vi "lvoption.vi"   [LabVIEW 2020]
uses:
  <vilib>/Wiresmith Technology/G CLI/Argument Parser/Option Class/Option Configuration.ctl
  <vilib>/Wiresmith Technology/G CLI/Argument Parser/Option Class/Argument Type.ctl
  <vilib>/Utility/error.llb/DialogType.ctl
  094f6021-4ef8-4573-82ce-a7b4949f6c5c.vi
  35111923-3b9e-4c36-b72b-79289da6bcaf.vi
  0b828e9d-cbba-40c4-b017-a79c080be190.vi
  6795289f-0a04-455c-a499-a5e59a361415.vi
  <resource>/dialog/lvconfig.llb/LV Config Read String.vi
  <resource>/dialog/lvconfig.llb/LV Config Write String.vi
  <resource>/dialog/lvconfig.llb/LV Config Write Boolean.vi
  <resource>/dialog/lvconfig.llb/LV Config Write Numeric (I32).vi
  <vilib>/Comparison/Equal/Equal Functor/Equal Functor.lvclass
  <vilib>/Wiresmith Technology/G CLI/CLI Class/CLI.lvclass
  <vilib>/Wiresmith Technology/G CLI/Argument Parser/Option Set Class/Option Set.lvclass
  <vilib>/Wiresmith Technology/G CLI/Argument Parser/Option Class/Option.lvclass
  <resource>/dialog/lvconfig.llb/LV Config Write Color.vi
  <resource>/dialog/lvconfig.llb/LV Config Write Pathlist.vi
types:
  T1 = cluster{"VerboseMode":bool, "Operation":string, "Key":string}
  T2 = enum32{"Invalid", "Standard", "Closed", "Hidden", "Minimized", "Maximized"}
  T3 = typedef "Option Parser.lvlib/Option.lvclass/Option Configuration.ctl" = cluster{"Option Type":T4, "Option Labels":string[], "Key":string, "Description":string, "Required":bool, "Default Value":string}
  T4 = typedef "Option Parser.lvlib/Option.lvclass/Argument Type.ctl" = enum16{"flag", "value"}
  T5 = typedef "DialogType.ctl" = u16
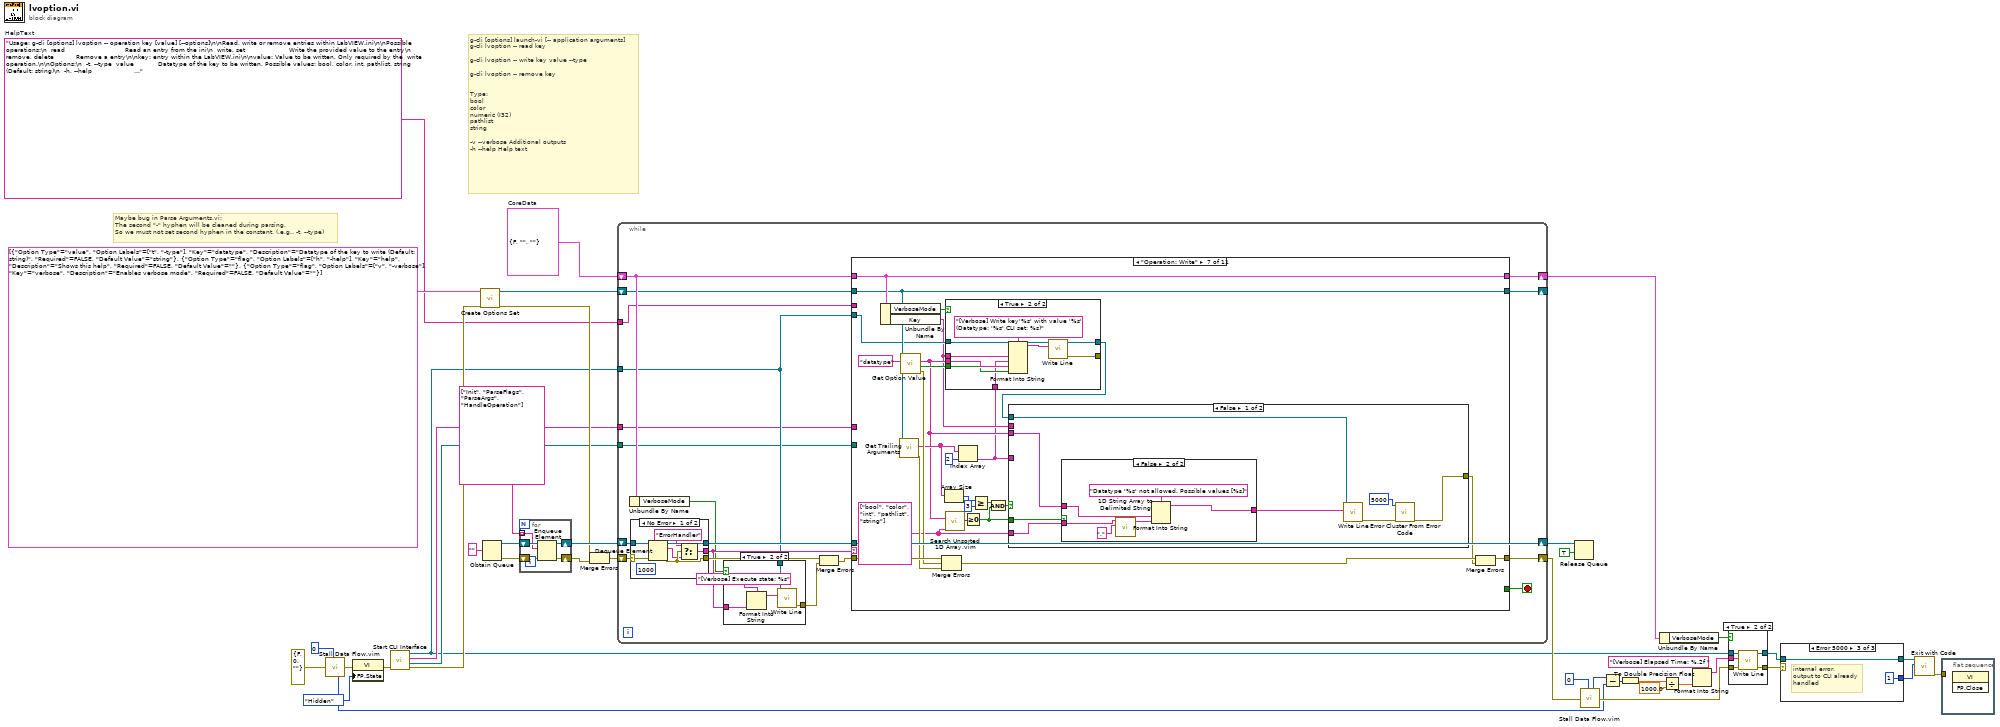
[diagram p0: block diagram]
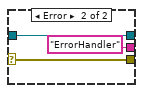
[diagram p4: hidden frame]
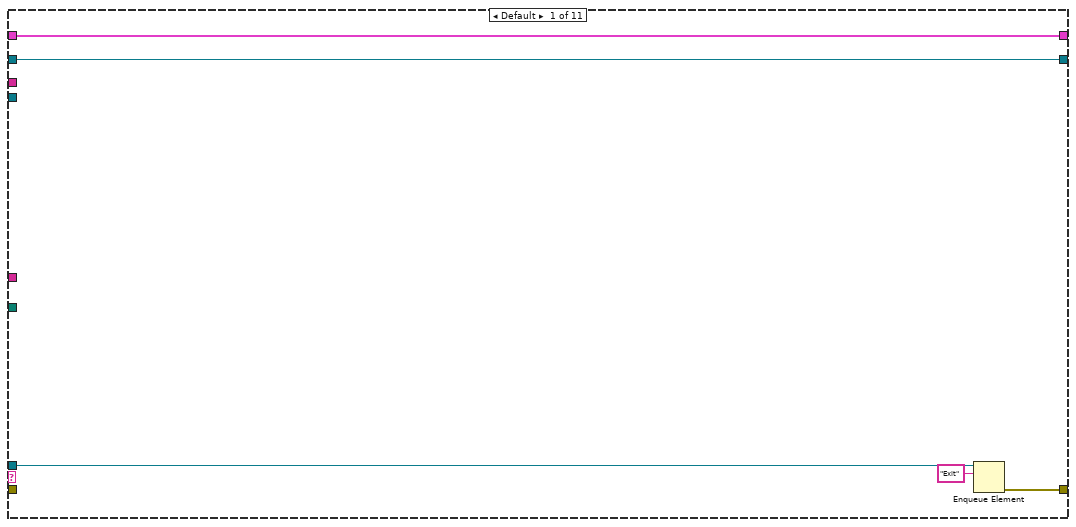
[diagram p5: hidden frame]
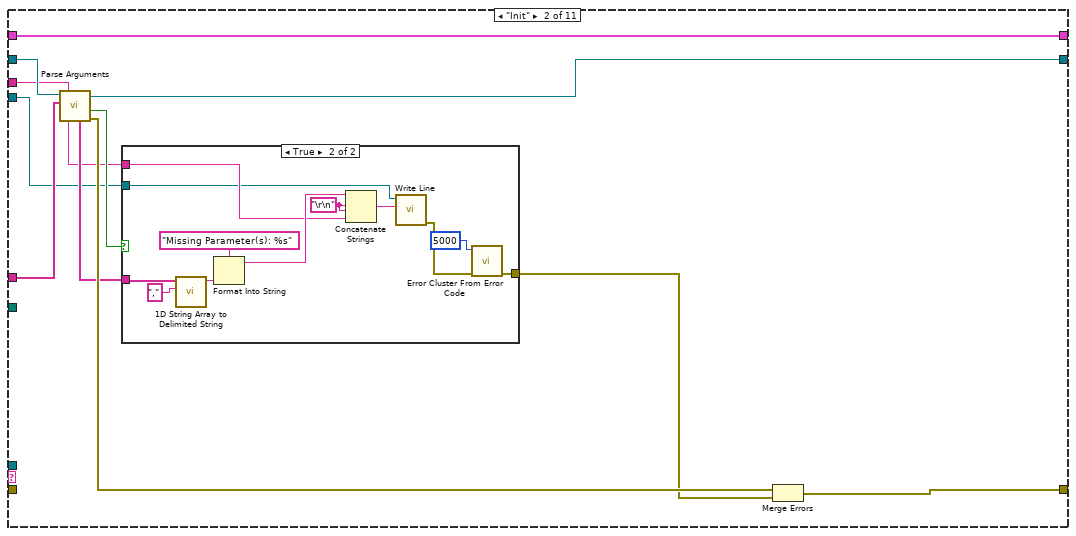
[diagram p6: hidden frame]
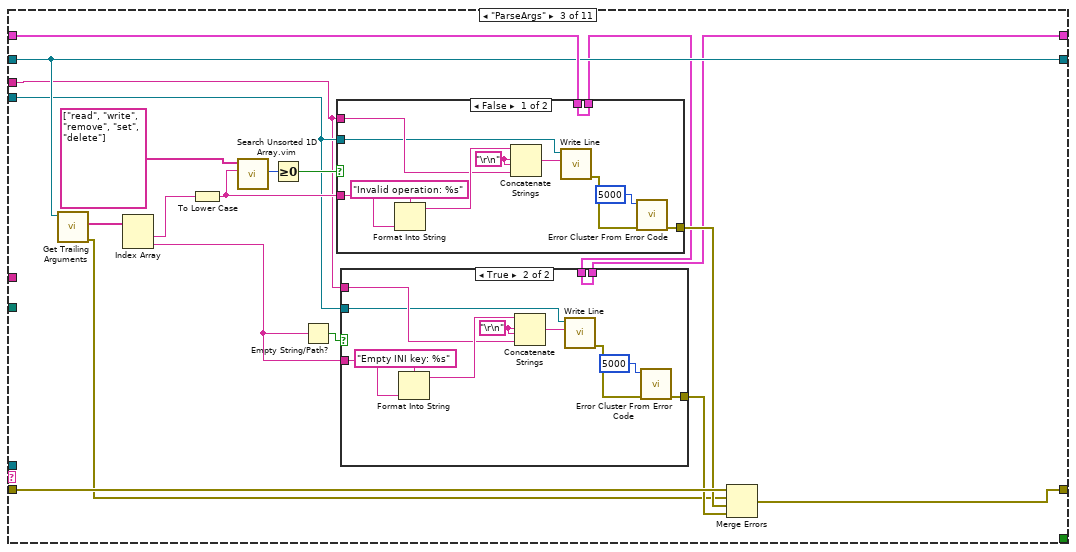
[diagram p8: hidden frame]
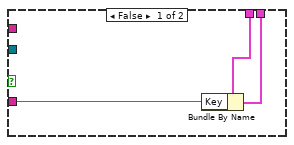
[diagram p9: hidden frame]
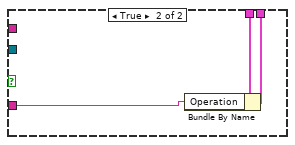
[diagram p10: hidden frame]
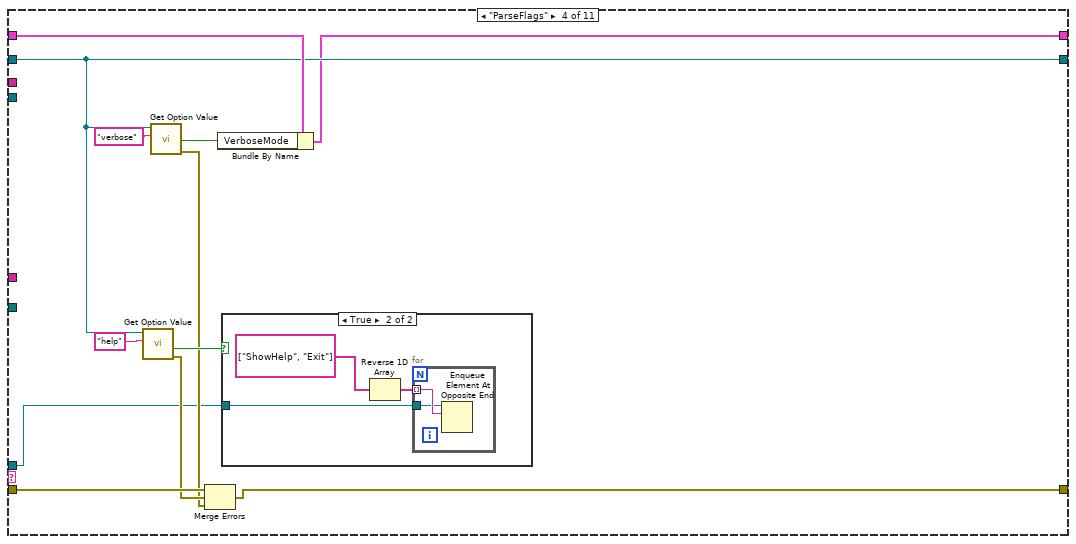
[diagram p11: hidden frame]
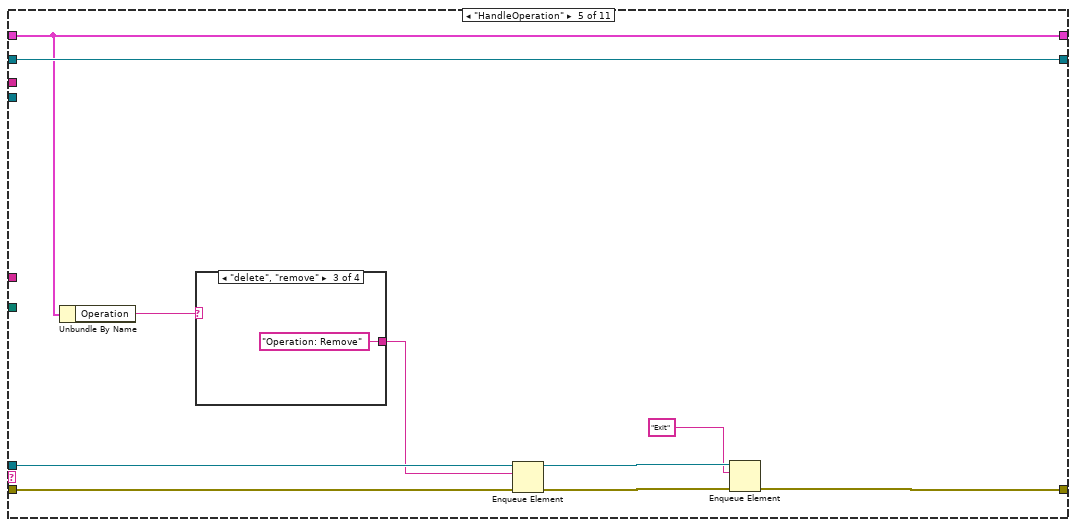
[diagram p13: hidden frame]
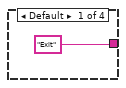
[diagram p14: hidden frame]
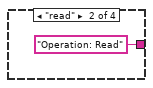
[diagram p15: hidden frame]
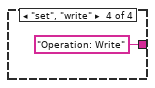
[diagram p16: hidden frame]
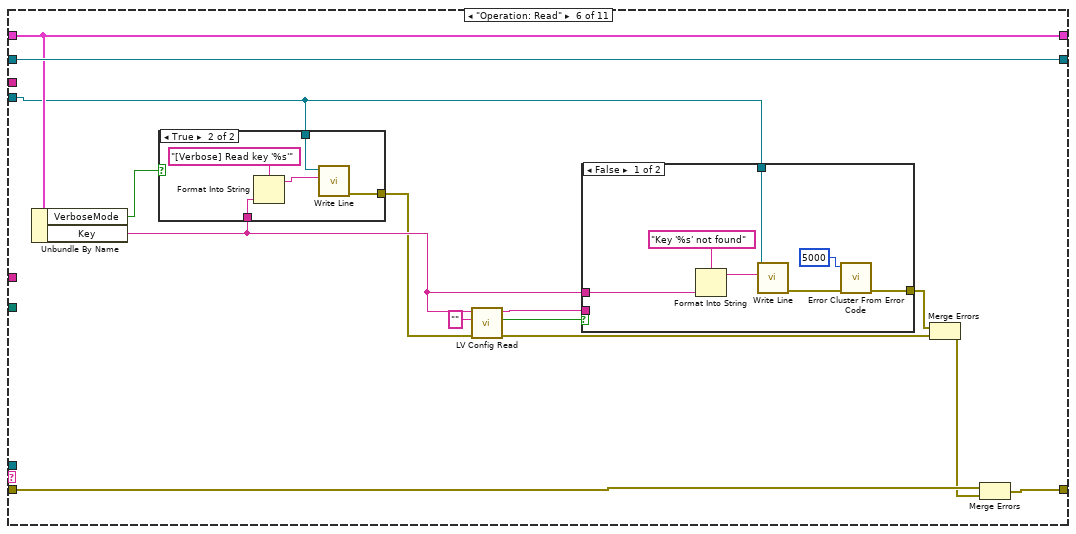
[diagram p17: hidden frame]
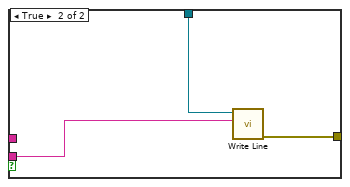
[diagram p19: hidden frame]
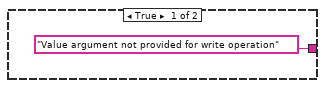
[diagram p20: hidden frame]
diagram:
  w1 = "Usage: g-cli [options] lvoption -- operation key [value] [--options]\n\nRead, write or remove entries within LabVIEW.ini\n\nPossible operations:\n  read                              Read an entry from the ini\n  write, set                      Write the provided value to the entry\n  remove, delete           Remove a entry\n\nkey: entry within the LabVIEW.ini\n\nvalue: Value to be written. Only required by the  write operation.\n\nOptions:\n  -t, --type  value            Datatype of the key to be written. Possible values: bool, color, int, pathlist, string (Default: string)\n  -h, --help                      Shows this help.\n  -v, --verbose                 Enables verbose mode."  # HelpText
  w14 = T1 {"VerboseMode"=FALSE, "Operation"="", "Key"=""}  # CoreData
  # "Maybe bug in Parse Arguments.vi: \nThe second \"-\" hyphen will be cleaned during parsing.\nSo we must not set second hyphen in the constant. (.e.g., -t, --type)"
  # "g-cli [options] launch-vi [-- application arguments]\ng-cli lvoption -- read key\n\ng-cli lvoption -- write key value --type \n\ng-cli lvoption -- remove key\n\n\nType:\nbool\ncolor\nnumeric (I32)\npathlist\nstring\n\n-v --verbose Additional outputs\n-h --help Help text"
  n1 = call "Stall Data Flow.vim"("value in"=errorcluster {"status"=FALSE, "code"=0, "source"=""} ("error in (no error)"), "milliseconds to wait"=u32 0) -> ("millisecond timer value"=w30:u32, "value out"=w37:errorcluster)
  n2 = property class="VI"(error in=w37, "FP.State"=T2."Hidden" ("Front Panel Window:State")) -> (error out=w36:errorcluster)  [unwired: 1 in, 1 out]
  n3 = call <vilib>:"Start CLI Interface.vi"("error in (no error)"=w36) -> ("error out"=w41:errorcluster, "Working Directory"=w7:path, "Custom Parameters"=w8:string[], "CLI out"=w5:refnum<class "CLI.lvclass">)  [unwired: 7 in]
  n4 = call <vilib>:"Create Options Set.vi"("error in (no error)"=w41, "Options"=T3[] [{"Option Type"=enum."value", "Option Labels"=["t", "-type"], "Key"="datatype", "Description"="Datatype of the key to write (Default: string)", "Required"=FALSE, "Default Value"="string"}, {"Option Type"=enum."flag", "Option Labels"=["h", "-help"], "Key"="help", "Description"="Shows this help", "Required"=FALSE, "Default Value"=""}, {"Option Type"=enum."flag", "Option Labels"=["v", "-verbose"], "Key"="verbose", "Description"="Enables verbose mode", "Required"=FALSE, "Default Value"=""}]) -> ("error out"=w10:errorcluster, "Option Set out"=w12:refnum<class "Option Set.lvclass">)  [unwired: 8 in]
  n5 = Obtain Queue(element data type="") -> (queue out=w19:refnum<queue>, error out=w16:errorcluster)  [unwired: 4 in, 1 out]
  n6 = for {
    shift-right: [w45] -> w17
    shift-left: w19 -> [w46]
    shift-right: [w43] -> w11
    shift-left: w16 -> [w44]
    tunnel: string[] ["Init", "ParseFlags", "ParseArgs", "HandleOperation"] -> [w42] mode=indexing
    n7 = Enqueue Element(queue=w46, element=w42, error in (no error)=w44) -> (queue out=w45:refnum<queue>, error out=w43:errorcluster)  [unwired: 1 in, 1 out]
  }
  n8 = Merge Errors(w10, w11) -> (w9:errorcluster)
  n9 = while {
    shift-right: [w61] -> w4
    shift-left: w14 -> [w56]
    shift-right: [w59] -> w6
    shift-left: w9 -> [w63]
    shift-right: [w58] -> w15
    shift-left: w17 -> [w64]
    tunnel: w5 -> [w54]
    tunnel: w8 -> [w49]
    tunnel: w7 -> [w50]
    tunnel: w1 -> [w48]
    shift-right: [w47] -> _
    shift-left: w12 -> [w53]
    stop <- w60 stop-if-true
    n10 = Unbundle By Name(w56) -> ("VerboseMode"=w55:bool)
    n11 = case shown="No Error" w63 {
      selector: w63 -> [w75 w79]
      tunnel: w64 -> [w76 w78]
      tunnel: [w71 "ErrorHandler"] -> w57
      tunnel: [w73 w79] -> w62
      tunnel: [w74 w78] -> w58
      frame No Error {
        (unwired) 1000 ("timeout in ms (-1)")
        n12 = Dequeue Element(queue=w76, error in (no error)=w75) -> (queue out=w74:refnum<queue>, element=w72:string, error out=w73:errorcluster)  [unwired: 1 in, 1 out]
        n13 = Select(t="ErrorHandler", s=w73, f=w72) -> (s? t:f=w71:string)
      }
      frame Error {
      }
    }
    n14 = case shown="True" w55 {
      tunnel: w57 -> [_ w69]
      tunnel: w54 -> [_ w66]
      tunnel: [_ w65] -> w51
      frame False {
      }
      frame True {
        n15 = Format Into String(format string="[Verbose] Execute state: %s", w69) -> (resulting string=w67:string)  [unwired: 2 in, 1 out]
        n16 = call <vilib>:"Write Line.vi"("Text to Write"=w67, "CLI in"=w66) -> ("error out"=w65:errorcluster)  [unwired: 8 in, 1 out]
      }
    }
    n17 = Merge Errors(w62, w51) -> (w52:errorcluster)
    n18 = case shown="\"Operation: Write\"" w57 {
      tunnel: w52 -> [_ _ w125 w163 w178 w197 w239 w300 _ w329 w332]
      tunnel: [w84 w95 w114 w155 w180 w198 w236 w305 w326 w330 w334] -> w61
      tunnel: w56 -> [w84 w95 w126 w166 w180 w198 w236 w305 w326 w330 w334]
      tunnel: [_ _ _ _ _ _ _ _ _ TRUE TRUE] -> w60
      tunnel: [w82 w87 w117 w160 w172 w196 w227 w307 w322 w329 w332] -> w59
      tunnel: w58 -> [w83 _ _ w156 w177 _ _ _ _ _ _]
      tunnel: w54 -> [_ w88 w113 _ _ w188 w224 w302 w324 _ _]
      tunnel: w53 -> [w80 w94 w124 w161 w181 w199 w234 w308 w325 w327 w331]
      tunnel: w50 -> [_ _ _ _ _ _ _ _ _ _ _]
      tunnel: w49 -> [_ w93 _ _ _ _ _ _ _ _ _]
      tunnel: w48 -> [_ w89 w112 _ _ _ _ _ w323 _ _]
      tunnel: [w80 w85 w124 w161 w181 w199 w234 w308 w325 w327 w331] -> w47
      frame Default {
        n19 = Enqueue Element(queue=w83, element="Exit") -> (error out=w82:errorcluster)  [unwired: 2 in, 2 out]
      }
      frame "Init" {
        n20 = call <vilib>:"Parse Arguments.vi"("Arguments"=w93, "Option Set in"=w94) -> ("error out"=w92:errorcluster, "Missing Options"=w91:bool, "Option Set out"=w85:refnum<class "Option Set.lvclass">, "Missing Option Keys"=w90:string[])  [unwired: 6 in]
        n21 = case shown="True" w91 {
          tunnel: w90 -> [_ w106]
          tunnel: w89 -> [_ w101]
          tunnel: w88 -> [_ w99]
          tunnel: [_ w96] -> w86
          frame False {
          }
          frame True {
            w103 = "\r\n"
            n22 = call <vilib>:"1D String Array to Delimited String.vi"("delimiter"=",", "string array"=w106) -> ("delimited string"=w104:string)  [unwired: 9 in]
            n23 = Format Into String(format string="Missing Parameter(s): %s", w104) -> (resulting string=w102:string)  [unwired: 2 in, 1 out]
            n24 = Concatenate Strings(w102, w103, w103, w101) -> (w100:string)
            n25 = call <vilib>:"Write Line.vi"("Text to Write"=w100, "CLI in"=w99) -> ("error out"=w97:errorcluster)  [unwired: 8 in, 1 out]
            n26 = call <vilib>:"Error Cluster From Error Code.vi"("error in (no error)"=w97, "error code (0)"=5000) -> ("error out"=w96:errorcluster)  [unwired: 7 in]
          }
        }
        n27 = Merge Errors(w92, w86) -> (w87:errorcluster)
      }
      frame "ParseArgs" {
        n28 = call <vilib>:"Get Trailing Arguments.vi"("Option Set in"=w124) -> ("error out"=w108:errorcluster, "Arguments"=w123:string[])  [unwired: 8 in, 1 out]
        n29 = Index Array(array=w123) -> (element #1=w122:string, element #2=w111:string)  [unwired: 2 in]
        n30 = To Lower Case(string=w122) -> (all lower case string=w118:string)
        n31 = call "Search Unsorted 1D Array.vim"("element"=w118, "unsorted 1D array"=string[] ["read", "write", "remove", "set", "delete"]) -> ("index of element"=w120:i32)  [unwired: 9 in]
        n32 = Greater Or Equal To 0?(x=w120) -> (x >= 0?=w119:bool)
        n33 = Empty String/Path?(string/path=w111) -> (empty?=w110:bool)
        n34 = case shown="False" w119 {
          tunnel: w112 -> [w148 _]
          tunnel: w113 -> [w146 _]
          tunnel: [w143 _] -> w116
          tunnel: w126 -> [w142 w154]
          tunnel: w118 -> [w141 w153]
          tunnel: [w142 w152] -> w115
          frame False {
            w150 = "\r\n"
            n35 = Format Into String(format string="Invalid operation: %s", w141) -> (resulting string=w149:string)  [unwired: 2 in, 1 out]
            n36 = Concatenate Strings(w149, w150, w150, w148) -> (w147:string)
            n37 = call <vilib>:"Write Line.vi"("Text to Write"=w147, "CLI in"=w146) -> ("error out"=w144:errorcluster)  [unwired: 8 in, 1 out]
            n38 = call <vilib>:"Error Cluster From Error Code.vi"("error in (no error)"=w144, "error code (0)"=5000) -> ("error out"=w143:errorcluster)  [unwired: 7 in]
          }
          frame True {
            n39 = Bundle By Name(cluster=w154, "Operation"=w153) -> (w152:T1)
          }
        }
        n40 = case shown="True" w110 {
          tunnel: w112 -> [_ w137]
          tunnel: w113 -> [_ w135]
          tunnel: [_ w132] -> w109
          tunnel: w115 -> [w129 w131]
          tunnel: w111 -> [w128 w130]
          tunnel: [w127 w131] -> w114
          frame False {
            n41 = Bundle By Name(cluster=w129, "Key"=w128) -> (w127:T1)
          }
          frame True {
            w139 = "\r\n"
            n42 = Format Into String(format string="Empty INI key: %s", w130) -> (resulting string=w138:string)  [unwired: 2 in, 1 out]
            n43 = Concatenate Strings(w138, w139, w139, w137) -> (w136:string)
            n44 = call <vilib>:"Write Line.vi"("Text to Write"=w136, "CLI in"=w135) -> ("error out"=w133:errorcluster)  [unwired: 8 in, 1 out]
            n45 = call <vilib>:"Error Cluster From Error Code.vi"("error in (no error)"=w133, "error code (0)"=5000) -> ("error out"=w132:errorcluster)  [unwired: 7 in]
          }
        }
        n46 = Merge Errors(w125, w108, w116, w109) -> (w117:errorcluster)
      }
      frame "ParseFlags" {
        n47 = call <vilib>:"Get Option Value.vi"("Option Key"="help", "Option Set in"=w161) -> ("error out"=w159:errorcluster, "Set"=w164:bool)  [unwired: 6 in, 2 out]
        n48 = call <vilib>:"Get Option Value.vi"("Option Key"="verbose", "Option Set in"=w161) -> ("error out"=w158:errorcluster, "Set"=w157:bool)  [unwired: 6 in, 2 out]
        n49 = Merge Errors(w163, w159, w158) -> (w160:errorcluster)
        n50 = Bundle By Name(cluster=w166, "VerboseMode"=w157) -> (w155:T1)
        n51 = case shown="True" w164 {
          tunnel: w156 -> [_ w168]
          frame False {
          }
          frame True {
            n52 = Reverse 1D Array(array=string[] ["ShowHelp", "Exit"]) -> (reversed array=w167:string[])
            n53 = for {
              tunnel: w167 -> [w171] mode=indexing
              tunnel: w168 -> [w170]
              n54 = Enqueue Element At Opposite End(queue=w170, element=w171) -> ()  [unwired: 2 in, 3 out]
            }
          }
        }
      }
      frame "HandleOperation" {
        n55 = Unbundle By Name(w180) -> ("Operation"=w179:string)
        n56 = case shown="\"delete\", \"remove\"" w179 {
          tunnel: ["Exit" "Operation: Read" "Operation: Remove" "Operation: Write"] -> w176
          frame Default {
          }
          frame "read" {
          }
          frame "delete", "remove" {
          }
          frame "set", "write" {
          }
        }
        n57 = Enqueue Element(queue=w177, element=w176, error in (no error)=w178) -> (queue out=w174:refnum<queue>, error out=w175:errorcluster)  [unwired: 1 in, 1 out]
        n58 = Enqueue Element(queue=w174, element="Exit", error in (no error)=w175) -> (error out=w172:errorcluster)  [unwired: 1 in, 2 out]
      }
      frame "Operation: Read" {
        n59 = Unbundle By Name(w198) -> ("VerboseMode"=w189:bool, "Key"=w187:string)
        n60 = case shown="True" w189 {
          tunnel: w188 -> [_ w204]
          tunnel: w187 -> [_ w201]
          tunnel: [_ w200] -> w186
          frame False {
          }
          frame True {
            n61 = Format Into String(format string="[Verbose] Read key '%s'", w201) -> (resulting string=w203:string)  [unwired: 2 in, 1 out]
            n62 = call <vilib>:"Write Line.vi"("Text to Write"=w203, "CLI in"=w204) -> ("error out"=w200:errorcluster)  [unwired: 8 in, 1 out]
          }
        }
        n63 = call-poly <resource>:"LV Config Read.vi"("error in"=w186, "default value"="", "key"=w187) -> ("error out"=w195:errorcluster, "found?"=w193:bool, "value"=w190:string)  [unwired: 2 in]
        n64 = case shown="False" w193 {
          tunnel: w187 -> [w207 _]
          tunnel: [w206 w213] -> w191
          tunnel: w188 -> [w205 w214]
          tunnel: w190 -> [_ w212]
          frame False {
            n65 = Format Into String(format string="Key '%s' not found", w207) -> (resulting string=w209:string)  [unwired: 2 in, 1 out]
            n66 = call <vilib>:"Write Line.vi"("Text to Write"=w209, "CLI in"=w205) -> ("error out"=w210:errorcluster)  [unwired: 8 in, 1 out]
            n67 = call <vilib>:"Error Cluster From Error Code.vi"("error in (no error)"=w210, "error code (0)"=5000) -> ("error out"=w206:errorcluster)  [unwired: 7 in]
          }
          frame True {
            n68 = call <vilib>:"Write Line.vi"("Text to Write"=w212, "CLI in"=w214) -> ("error out"=w213:errorcluster)  [unwired: 8 in, 1 out]
          }
        }
        n69 = Merge Errors(w191, w195) -> (w192:errorcluster)
        n70 = Merge Errors(w197, w192) -> (w196:errorcluster)
      }
      frame "Operation: Write" {
        w218 = string[] ["bool", "color", "int", "pathlist", "string"]
        n71 = Unbundle By Name(w236) -> ("VerboseMode"=w235:bool, "Key"=w216:string)
        n72 = call <vilib>:"Get Trailing Arguments.vi"("Option Set in"=w234) -> ("error out"=w230:errorcluster, "Arguments"=w228:string[])  [unwired: 8 in, 1 out]
        n73 = call <vilib>:"Get Option Value.vi"("Option Key"="datatype", "Option Set in"=w234) -> ("error out"=w229:errorcluster, "Set"=w237:bool, "Value"=w221:string)  [unwired: 6 in, 1 out]
        n74 = Merge Errors(w239, w229, w230) -> (w231:errorcluster)
        n75 = Array Size(array=w228) -> (size(s)=w233:i32)
        n76 = call "Search Unsorted 1D Array.vim"("element"=w221, "unsorted 1D array"=w218) -> ("index of element"=w222:i32)  [unwired: 9 in]
        n77 = Index Array(array=w228, index=2) -> (element=w215:string)
        n78 = case shown="True" w235 {
          tunnel: w221 -> [_ w299]
          tunnel: w237 -> [_ w298]
          tunnel: w224 -> [w290 w295]
          tunnel: [w290 w294] -> w225
          tunnel: [_ w293] -> _
          tunnel: w216 -> [_ w292]
          tunnel: w215 -> [_ w291]
          frame False {
          }
          frame True {
            n79 = Format Into String(format string="[Verbose] Write key'%s' with value '%s' (Datatype: '%s' CLI set: %s)", w292, w291, w299, w298) -> (resulting string=w296:string)  [unwired: 2 in, 1 out]
            n80 = call <vilib>:"Write Line.vi"("Text to Write"=w296, "CLI in"=w295) -> ("error out"=w293:errorcluster, "CLI out"=w294:refnum<class "CLI.lvclass">)  [unwired: 8 in]
          }
        }
        n81 = Greater Or Equal To 0?(x=w222) -> (x >= 0?=w220:bool)
        n82 = Greater Or Equal?(x=w233, y=3) -> (x >= y?=w219:bool)
        n83 = Compound Arithmetic op=AND(w219, w220) -> (w223:bool)
        n84 = case shown="False" w223 {
          tunnel: w225 -> [w244 w256]
          tunnel: [w243 w257] -> w226
          tunnel: w221 -> [w241 w258]
          tunnel: w220 -> [w242 _]
          tunnel: w218 -> [w240 _]
          tunnel: w216 -> [_ w259]
          tunnel: w215 -> [_ w255]
          frame False {
            n85 = case shown="False" w242 {
              tunnel: ["Value argument not provided for write operation" ("format string") w254] -> w245
              tunnel: w241 -> [_ w252]
              tunnel: w240 -> [_ w251]
              frame True {
              }
              frame False {
                n86 = call <vilib>:"1D String Array to Delimited String.vi"("delimiter"=",", "string array"=w251) -> ("delimited string"=w249:string)  [unwired: 9 in]
                n87 = Format Into String(format string="Datatype '%s' not allowed. Possible values [%s]", w252, w249) -> (resulting string=w254:string)  [unwired: 2 in, 1 out]
              }
            }
            n88 = call <vilib>:"Write Line.vi"("Text to Write"=w245, "CLI in"=w244) -> ("error out"=w246:errorcluster)  [unwired: 8 in, 1 out]
            n89 = call <vilib>:"Error Cluster From Error Code.vi"("error in (no error)"=w246, "error code (0)"=5000) -> ("error out"=w243:errorcluster)  [unwired: 7 in]
          }
          frame True {
            n90 = case shown="\"string\", Default" w258 {
              tunnel: w259 -> [w261 w265 w271 w274 w284]
              tunnel: [w262 w266 w270 w273 w283] -> w257
              tunnel: w256 -> [_ _ _ w272 _]
              tunnel: w255 -> [w260 w263 w269 _ w282]
              frame "string", Default {
                n91 = call-poly <resource>:"LV Config Write.vi"("value"=w260, "key"=w261) -> ("error out"=w262:errorcluster)  [unwired: 5 in]
              }
              frame "bool" {
                n92 = case shown="\"0\", \"disable\", \"disabled\", \"False\", \"off\", Default" w263 {
                  tunnel: [_ TRUE] -> w264
                  frame "0", "disable", "disabled", "False", "off", Default {
                  }
                  frame "1", "enable", "enabled", "on", "True" {
                  }
                }
                n93 = call-poly <resource>:"LV Config Write.vi"("value"=w264, "key"=w265) -> ("error out"=w266:errorcluster)  [unwired: 5 in]
              }
              frame "int" {
                n94 = Decimal String To Number(string=w269) -> (number=w268:i32)  [unwired: 2 in, 1 out]
                n95 = call-poly <resource>:"LV Config Write.vi"("value"=w268, "key"=w271) -> ("error out"=w270:errorcluster)  [unwired: 5 in]
              }
              frame "color" {
                n96 = disable-structure shown="Enabled" {
                  disable-tunnel: w274 -> [w276 _]
                  disable-tunnel: [w275 w278] -> w273
                  disable-tunnel: w272 -> [_ w277]
                  frame Disabled {
                    n97 = call-poly <resource>:"LV Config Write.vi"("key"=w276) -> ("error out"=w275:errorcluster)  [unwired: 6 in]
                  }
                  frame Enabled {
                    n98 = call <vilib>:"Write Line.vi"("Text to Write"="Operation 'Write' for datatype 'color' not implemented" ("format string"), "CLI in"=w277) -> ("error out"=w280:errorcluster)  [unwired: 8 in, 1 out]
                    n99 = call <vilib>:"Error Cluster From Error Code.vi"("error in (no error)"=w280, "error code (0)"=5000) -> ("error out"=w278:errorcluster)  [unwired: 7 in]
                  }
                }
              }
              frame "pathlist" {
                n100 = disable-structure shown="Enabled" {
                  disable-tunnel: w284 -> [w286 w288]
                  disable-tunnel: [w285 w287] -> w283
                  disable-tunnel: w282 -> [_ w289]
                  frame Disabled {
                    n101 = call-poly <resource>:"LV Config Write.vi"("key"=w286) -> ("error out"=w285:errorcluster)  [unwired: 6 in]
                  }
                  frame Enabled {
                    # "do not convert value: list must be separated by ';' semi-colon"
                    n102 = call-poly <resource>:"LV Config Write.vi"("value"=w289, "key"=w288) -> ("error out"=w287:errorcluster)  [unwired: 5 in]
                  }
                }
              }
            }
          }
        }
        n103 = Merge Errors(w231, w226) -> (w227:errorcluster)
      }
      frame "Operation: Remove" {
        n104 = Unbundle By Name(w305) -> ("VerboseMode"=w306:bool, "Key"=w304:string)
        n105 = case shown="True" w306 {
          tunnel: w302 -> [_ w321]
          tunnel: w304 -> [_ w318]
          tunnel: [_ w317] -> w303
          frame False {
          }
          frame True {
            n106 = Format Into String(format string="[Verbose] Remove key '%s'", w318) -> (resulting string=w320:string)  [unwired: 2 in, 1 out]
            n107 = call <vilib>:"Write Line.vi"("Text to Write"=w320, "CLI in"=w321) -> ("error out"=w317:errorcluster)  [unwired: 8 in, 1 out]
          }
        }
        n108 = disable-structure shown="Enabled" {
          disable-tunnel: w304 -> [w311 _]
          disable-tunnel: w303 -> [w310 _]
          disable-tunnel: w302 -> [_ w313]
          disable-tunnel: [w309 w312] -> w301
          frame Enabled {
            n109 = call <resource>:"LV Config Remove.vi"("error in"=w310, "key"=w311) -> ("error out"=w309:errorcluster)  [unwired: 5 in]
          }
          frame Disabled {
            n110 = call <vilib>:"Write Line.vi"("Text to Write"="Operation 'Remove' not implemented" ("format string"), "CLI in"=w313) -> ("error out"=w316:errorcluster)  [unwired: 8 in, 1 out]
            n111 = call <vilib>:"Error Cluster From Error Code.vi"("error in (no error)"=w316, "error code (0)"=5000) -> ("error out"=w312:errorcluster)  [unwired: 7 in]
          }
        }
        n112 = Merge Errors(w300, w301) -> (w307:errorcluster)
      }
      frame "ShowHelp" {
        n113 = call <vilib>:"Write Line.vi"("Text to Write"=w323, "CLI in"=w324) -> ("error out"=w322:errorcluster)  [unwired: 8 in, 1 out]
      }
      frame "ErrorHandler" {
      }
      frame "Exit" {
      }
    }
  }
  n114 = Release Queue(queue=w15, force destroy? (F)=TRUE) -> ()  [unwired: 1 in, 3 out]
  n115 = call "Stall Data Flow.vim"("value in"=w6, "milliseconds to wait"=u32 0) -> ("millisecond timer value"=w31:u32, "value out"=w39:errorcluster)
  n116 = Subtract(x=w31, y=w30) -> (x-y=w29:u32)
  n117 = To Double Precision Float(number=w29) -> (double precision float=w28:dbl)
  n118 = Unbundle By Name(w4) -> ("VerboseMode"=w3:bool)
  n119 = Divide(x=w28, y=1000.0) -> (x/y=w26:dbl)
  n120 = Format Into String(format string="[Verbose] Elapsed Time: %.2f ", w26) -> (resulting string=w24:string)  [unwired: 2 in, 1 out]
  n121 = case shown="True" w3 {
    tunnel: w39 -> [w335 w341]
    tunnel: [w335 w340] -> w38
    tunnel: w5 -> [w336 w339]
    tunnel: w24 -> [_ w338]
    tunnel: [w336 w337] -> w23
    frame False {
    }
    frame True {
      n122 = call <vilib>:"Write Line.vi"("error in (no error)"=w341, "Text to Write"=w338, "CLI in"=w339) -> ("error out"=w340:errorcluster, "CLI out"=w337:refnum<class "CLI.lvclass">)  [unwired: 7 in]
    }
  }
  n123 = case shown="Error 5000" w38 {
    selector: w38 -> [_ w348 _]
    tunnel: w23 -> [w342 w347 w349]
    tunnel: [w342 w346 w349] -> w22
    tunnel: [_ w343 1 ("code out")] -> w21
    frame No Error {
    }
    frame Default {
      w345 = T5 0 items=["no dialog", "OK message", "continue or stop message", "OK message + warnings", "continue/stop + warnings"] ("type of dialog (OK msg:1)")
      n124 = call <vilib>:"Simple Error Handler.vi"("type of dialog (OK msg:1)"=w345, "error in (no error)"=w348) -> ("code out"=w343:i32, "message"=w344:string)  [unwired: 3 in, 3 out]
      n125 = call <vilib>:"Write Line.vi"("Text to Write"=w344, "CLI in"=w347) -> ("CLI out"=w346:refnum<class "CLI.lvclass">)  [unwired: 8 in, 1 out]
    }
    frame Error {
      # "internal error, \noutput to CLI already\nhandled"
    }
  }
  n126 = call <vilib>:"Exit with Code.vi"("Exit Code (0)"=w21, "CLI in"=w22) -> ("error out"=w35:errorcluster)  [unwired: 9 in]
  n127 = flat-sequence {
    tunnel: w35 -> [_]
    frame #0 {
      n128 = invoke class="VI" method="FP.Close"() -> ()  [unwired: 3 in, 3 out]
    }
  }
